vi "Get Dilution Data.vi"(8 "error in (no error)":errorcluster, 10 "Complete NMEA Sentences":string[](array[string]), 11 "VISA resource name":refnum<visa-resource-name>) -> (0 "error out":errorcluster, 1 "Dilution Data":T1(array[cluster]), 2 "Complete NMEA Sentences (Copy)":string[](array[string]), 3 "VISA resource name out":refnum<visa-resource-name>)   [LabVIEW 2009]
doc: "Parses out the dilution data from all of the sentences that Read Raw.vi outputs, and passes through a complete copy of those sentences. Can be used in conjunction with other advanced \"Get\" VIs. See u-blox 5 Series Acquire and Chart GPS Advanced.vi for an example of how to use this VI.\n\nNote that the VISA Resource is not required, since this VI is a helper that does not actually interact with the device. The VISA Resource can be used, however, to clarify programming and maintain uniformity."
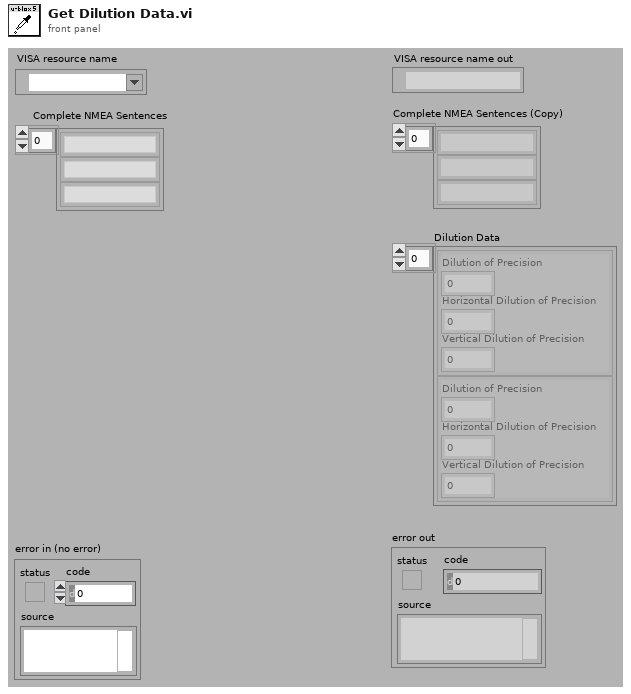
[diagram p1: front panel]
types:
  T1 = cluster{"Dilution of Precision":dbl, "Horizontal Dilution of Precision":dbl, "Vertical Dilution of Precision":dbl}[]
  T2 = cluster{"Dilution of Precision":dbl, "Horizontal Dilution of Precision":dbl, "Vertical Dilution of Precision":dbl}
  T3 = typedef "GSA Data.ctl" = cluster{"selection of fix":cluster{"included?":bool, "selection of 2D or 3D fix":u16}, "type of fix":cluster{"included?":bool, "mode":u16}, "satellite PRN numbers":cluster{"included?":bool[], "PRN numbers":i32[]}, "dilution of precision":cluster{"included?":bool, "DOP":dbl}, "horizontal dilution of precision":cluster{"included?":bool, "horizontal DOP":dbl}, "vertical dilution of precision":cluster{"included?":bool, "vertical DOP":dbl}}
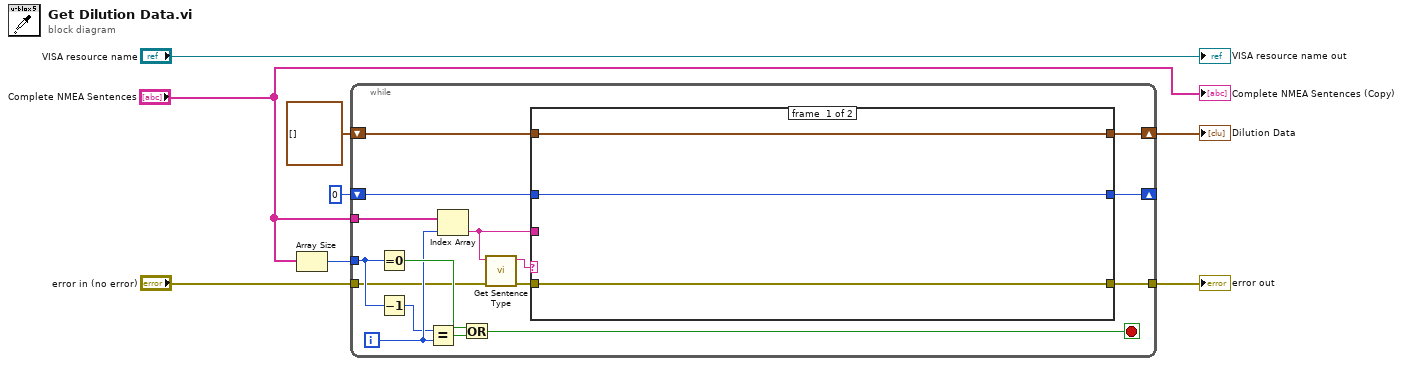
[diagram p0: block diagram]
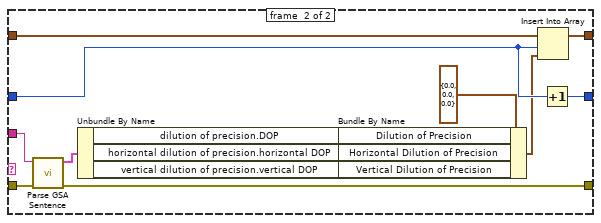
[diagram p2: hidden frame]
diagram:
  n1 = Array Size(array="Complete NMEA Sentences") -> (size(s)=w7:i32)
  n2 = while {
    tunnel: "Complete NMEA Sentences" -> [w24]
    shift-right: [w22] -> w1
    shift-left: T1 [] -> [w21]
    tunnel: w7 -> [w18]
    tunnel: "error in (no error)" -> [w11]
    tunnel: [w23] -> w5
    shift-right: [w19] -> _
    shift-left: 0 -> [w20]
    i -> [w14]
    stop <- w16 stop-if-true
    n3 = Equal To 0?(x=w18) -> (x = 0?=w17:bool)
    n4 = Decrement(x=w18) -> (x-1=w13:i32)
    n5 = Equal?(x=w13, y=w14) -> (x = y?=w15:bool)
    n6 = Index Array(array=w24, index=w14) -> (element=w9:string)
    n7 = Or(x=w17, y=w15) -> (x .or. y?=w16:bool)
    n8 = call "Get Sentence Type.vi"("error in (no error)"=w11, "sentence"=w9) -> ("error out"=w12:errorcluster, "sentence type"=w10:string)  [unwired: 7 in, 1 out]
    n9 = case shown="\"\", Default" w10 {
      tunnel: w9 -> [_ w29]
      tunnel: w12 -> [w27 w28]
      tunnel: [w27 w31] -> w23
      tunnel: [w26 w40] -> w22
      tunnel: w21 -> [w26 w39]
      tunnel: w20 -> [w25 w34]
      tunnel: [w25 w38] -> w19
      frame #0 {
      }
      frame #1 {
        n10 = call "Parse GSA Sentence.vi"("error in (no error)"=w28, "GSA sentence"=w29) -> ("error out"=w31:errorcluster, "GSA data"=w30:T3)  [unwired: 8 in]
        n11 = Unbundle By Name(w30) -> ("dilution of precision.DOP"=w35:dbl, "horizontal dilution of precision.horizontal DOP"=w36:dbl, "vertical dilution of precision.vertical DOP"=w33:dbl)
        n12 = Bundle By Name(cluster=T2 {"Dilution of Precision"=0.0, "Horizontal Dilution of Precision"=0.0, "Vertical Dilution of Precision"=0.0}, "Dilution of Precision"=w35, "Horizontal Dilution of Precision"=w36, "Vertical Dilution of Precision"=w33) -> (w32:T2)
        n13 = Insert Into Array(array=w39, index=w34, new element=w32) -> (w40:T1)
        n14 = Increment(x=w34) -> (x+1=w38:i32)
      }
    }
  }
  "error out" <- w5
  "Dilution Data" <- w1
  "VISA resource name out" <- "VISA resource name"
  "Complete NMEA Sentences (Copy)" <- "Complete NMEA Sentences"
